vi "onRemoveHeader.vi"(8 "error in":errorcluster, 10 "header":string, 11 "basic-http-client in":refnum<class "basic-http-client.lvclass">) -> (0 "error out":errorcluster, 3 "basic-http-client out":refnum<class "basic-http-client.lvclass">)   [LabVIEW 2020, in "REST Client.lvlib" / "basic-http-client.lvclass"]
uses:
  basic-http-client.lvclass
  basic-http-client.lvclass/basic-http-client.ctl
  <vilib>/httpClient/LabVIEWHTTPClient.lvlib
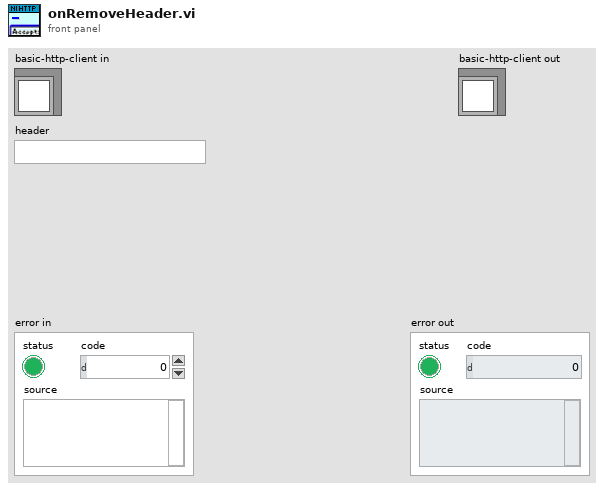
[diagram p1: front panel]
types:
  T1 = typedef "LabVIEWHTTPClient.lvlib/ClientHandle.ctl" = refnum<k1>
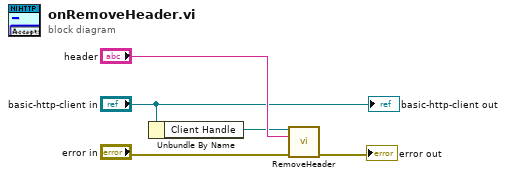
[diagram p0: block diagram]
diagram:
  n1 = Unbundle By Name("basic-http-client in") -> ("Client Handle"=w1:T1)
  n2 = call <vilib>:"RemoveHeader.vi"("client handle"=w1, "header"="header", "error in (no error)"="error in") -> ("error out"=→"error out":errorcluster)  [unwired: 11 in, 1 out]
  "basic-http-client out" <- "basic-http-client in"
